vi "Enq_Save_QMH.vi"(6 "Priority?":bool, 8 "Error In":errorcluster, 9 "Message":variant, 10 "Instruction":T1, 11 "Queue In":refnum<queue>) -> (0 "Error Out":errorcluster, 3 "Queue Out":refnum<queue>)   [LabVIEW 2021, in "Queues.lvlib"]
doc: "This subVI is used to budle and queue the elements in the Save QMH queue."
uses:
  Queues.lvlib
  Tipski Definicii/Save_Sostojbi.ctl
panel:
  # "Input"
  # "Output"
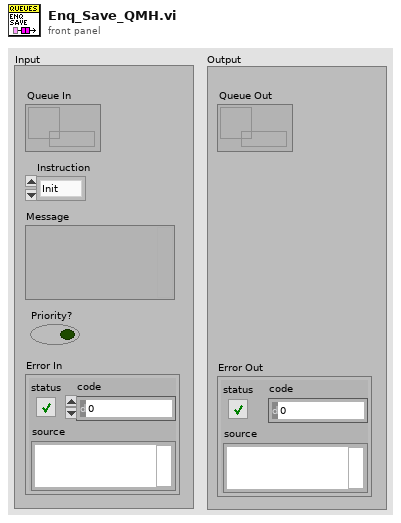
[diagram p1: front panel]
types:
  T1 = typedef "Save_Sostojbi.ctl" = enum16{"Init", "Generate Message", "Pick Path", "Save", "End"}
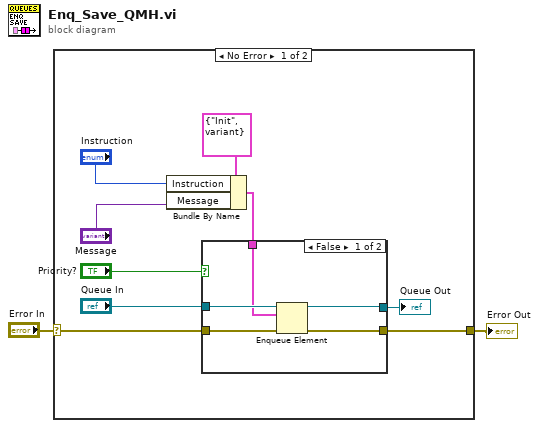
[diagram p0: block diagram]
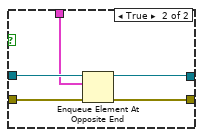
[diagram p2: hidden frame]
diagram:
  n1 = case shown="No Error" "Error In" {
    selector: "Error In" -> [w9 w22]
    tunnel: [w7 w22] -> w1
    frame No Error {
      n2 = Bundle By Name(cluster=cluster{"Instruction":T1, "Message":variant} {"Instruction"=enum."Init", "Message"=variant} ("element"), "Instruction"="Instruction", "Message"="Message") -> (w8:cluster{"Instruction":T1, "Message":variant})
      n3 = case shown="False" "Priority?" {
        tunnel: "Queue In" -> [w16 w20]
        tunnel: w9 -> [w15 w21]
        tunnel: w8 -> [w12 w17]
        tunnel: [w14 w18] -> w5
        tunnel: [w13 w19] -> w7
        frame False {
          n4 = Enqueue Element(queue=w16, element=w12, error in (no error)=w15) -> (queue out=w14:refnum<queue>, error out=w13:errorcluster)  [unwired: 1 in, 1 out]
        }
        frame True {
          n5 = Enqueue Element At Opposite End(queue=w20, element=w17, error in (no error)=w21) -> (queue out=w18:refnum<queue>, error out=w19:errorcluster)  [unwired: 1 in, 1 out]
        }
      }
      "Queue Out" <- w5
    }
    frame Error {
    }
  }
  "Error Out" <- w1
